vi "Set Inline.vi"(10 "inline":bool, 11 "Transfer Group in":refnum<class "Transfer Group.lvclass">) -> (3 "Transfer Group out":refnum<class "Transfer Group.lvclass">)   [LabVIEW 2019, in "DSF Core.lvlib" / "Transfer Group.lvclass"]
uses:
  Transfer Group.lvclass
  Transfer Group.lvclass/Transfer Group.ctl
  Transfer/Transfer.lvclass
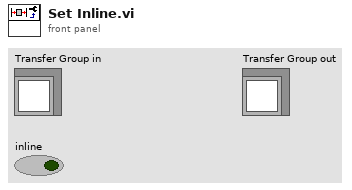
[diagram p1: front panel]
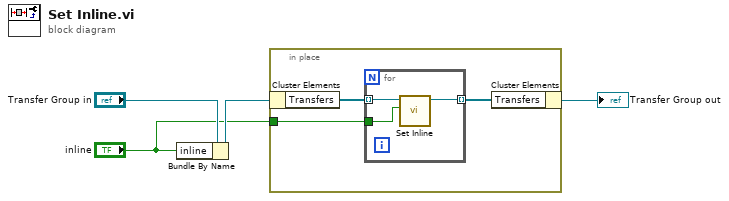
[diagram p0: block diagram]
diagram:
  n1 = Bundle By Name(cluster="Transfer Group in", "inline"="inline") -> (w3:refnum<class "Transfer Group.lvclass">)
  n2 = in-place {
    in-place-border: "inline" -> [w5]
    n3 = in-place-cluster #1(w3) -> ("Transfers"=w7:refnum<class "Transfer.lvclass">[])
    n4 = for {
      tunnel: w7 -> [w10] mode=indexing
      tunnel: [w9] -> w6 mode=indexing
      tunnel: w5 -> [w8]
      n5 = call "Set Inline.vi"("inline"=w8, "Transfer in"=w10) -> ("Transfer out"=w9:refnum<class "Transfer.lvclass">)  [unwired: 9 in]
    }
    n6 = in-place-cluster #1("Transfers"=w6) -> (→"Transfer Group out":refnum<class "Transfer Group.lvclass">)
  }
